vi "TSM DCPower Initialize Sessions.vi"(0 "TSM context":T2, 5 "Power Line Frequency":T1=60.0 caption="Power Line Frequency (60Hz)" items=["50 Hertz"=50.0, "60 Hertz"=60.0], 7 "Use Measure Multiple for Auto Measurement Mode? (T)":bool=TRUE) -> (15 "error out":errorcluster)   [LabVIEW 2020]
uses:
  <vilib>/NI_TestStand_SemiconductorModule/NI_TestStand_Semiconductor_Module.lvlibp/PinMap/General/SemiconductorModuleContext.ctl
  <instrlib>/niDCPower/nidcpower.llb/niDCPower Power Line Frequency.ctl
  <instrlib>/niDCPower/nidcpower.llb/niDCPower Sense.ctl
  SSC DCPower/Measure/SSC DCPower Debug Global.vi
  <vilib>/regexp/Match Regular Expression.xnode
  <vilib>/NI_TestStand_SemiconductorModule/NI_TestStand_Semiconductor_Module.lvlibp
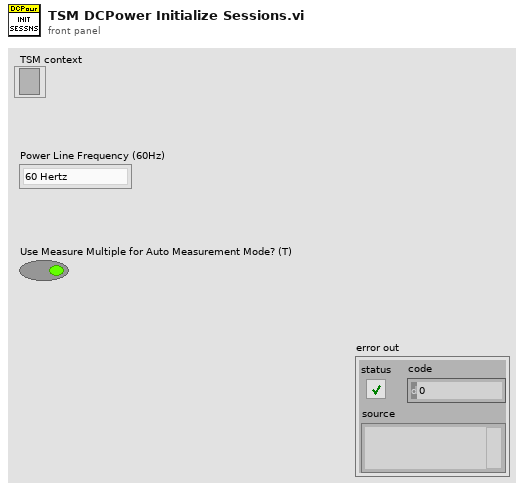
[diagram p1: front panel]
types:
  T1 = typedef "niDCPower Power Line Frequency.ctl" = dbl
  T2 = typedef "NI_TestStand_Semiconductor_Module.lvlibp/SemiconductorModuleContext.ctl" = refnum<k7>
  T3 = typedef "niDCPower Sense.ctl" = i32
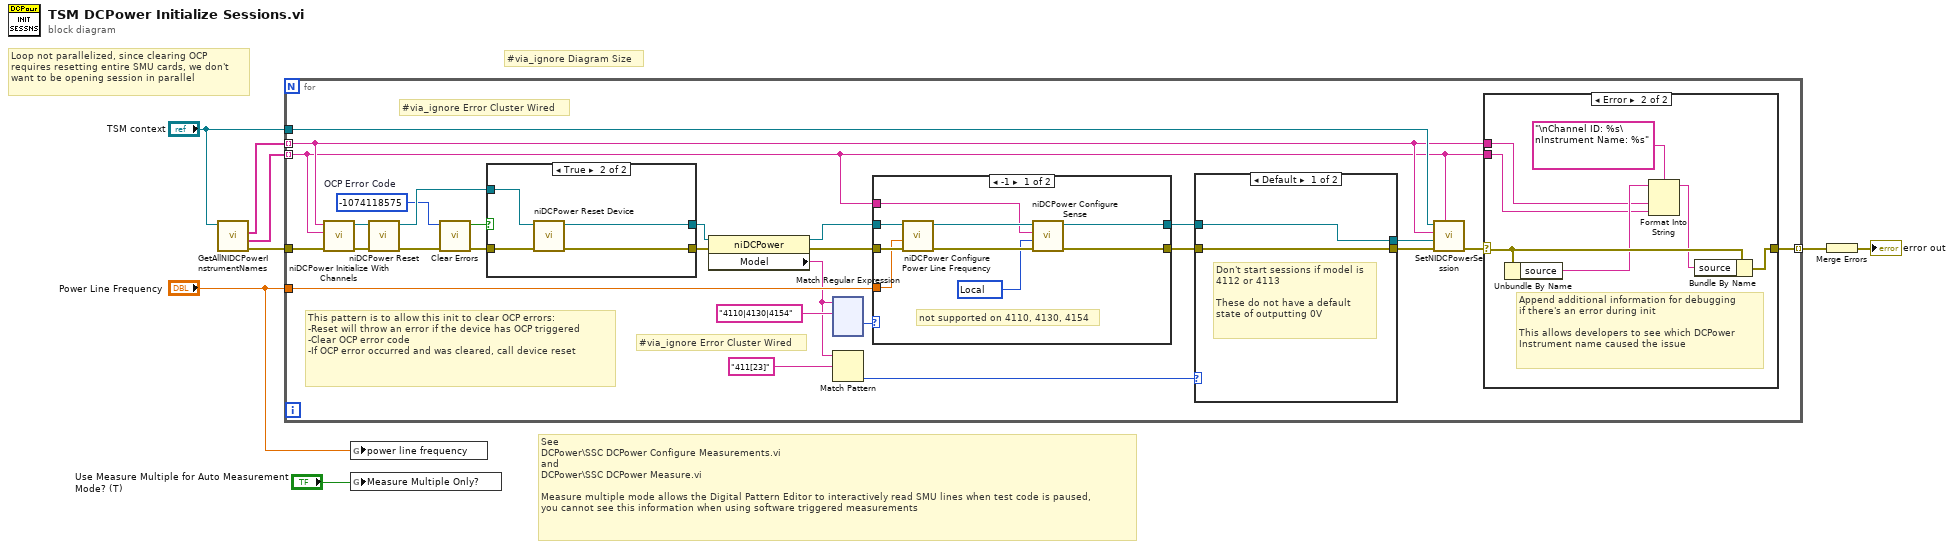
[diagram p0: block diagram]
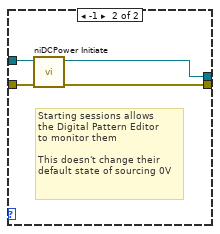
[diagram p5: hidden frame]
diagram:
  # "See \nDCPower\\SSC DCPower Configure Measurements.vi\nand\nDCPower\\SSC DCPower Measure.vi\n\nMeasure multiple mode allows the Digital Pattern Editor to interactively read SMU lines when test code is paused,\nyou cannot see this information when using software triggered measurements"
  # "#via_ignore Diagram Size"
  # "Loop not parallelized, since clearing OCP requires resetting entire SMU cards, we don't want to be opening session in parallel"
  n1 = call <vilib>:"GetAllNIDCPowerInstrumentNames.vi"("Semiconductor Module Context"="TSM context") -> ("error out"=w5:errorcluster, "Channel Ids"=w8:string[], "Instrument Names"=w4:string[])  [unwired: 7 in, 1 out]
  n2 = for {
    tunnel: w4 -> [w10] mode=indexing
    tunnel: w8 -> [w9] mode=indexing
    tunnel: "TSM context" -> [w35]
    tunnel: "Power Line Frequency" -> [w25]
    tunnel: w5 -> [w19]
    tunnel: [w11] -> w6 mode=indexing
    w14 = -1074118575  # OCP Error Code
    # "#via_ignore Error Cluster Wired"
    # "This pattern is to allow this init to clear OCP errors:\n-Reset will throw an error if the device has OCP triggered\n-Clear OCP error code\n-If OCP error occurred and was cleared, call device reset"
    # "#via_ignore Error Cluster Wired"
    n3 = call <instrlib>:"niDCPower Initialize With Channels.vi"("error in (no error)"=w19, "channels"=w9, "resource name"=w10) -> ("error out"=w31:errorcluster, "instrument handle out"=w17:refnum<k15>)  [unwired: 7 in]
    n4 = call <instrlib>:"niDCPower Reset.vi"("error in (no error)"=w31, "instrument handle"=w17) -> ("error out"=w18:errorcluster, "instrument handle out"=w16:refnum<k15>)  [unwired: 8 in]
    n5 = call <vilib>:"Clear Errors.vi"("error in (no error)"=w18, "specific error code to clear (0: all)"=w14) -> ("error out"=w15:errorcluster, "specific error cleared?"=w13:bool)  [unwired: 4 in]
    n6 = case shown="True" w13 {
      tunnel: [w44 w49] -> w21
      tunnel: w16 -> [w45 w46]
      tunnel: [w45 w48] -> w20
      tunnel: w15 -> [w44 w47]
      frame False {
      }
      frame True {
        n7 = call <instrlib>:"niDCPower Reset Device.vi"("error in (no error)"=w47, "instrument handle"=w46) -> ("error out"=w49:errorcluster, "instrument handle out"=w48:refnum<k15>)  [unwired: 8 in]
      }
    }
    n8 = property class="niDCPower"(reference=w20, error in=w21) -> (reference out=w27:refnum<k15>, error out=w30:errorcluster, "Model"=w22:string)
    n9 = xnode "Match Regular Expression"("input string"=w22, "regular expression"="4110|4130|4154") -> ("offset past match"=w23:i32)  [unwired: 4 in, 4 out]
    n10 = Match Pattern(string=w22, regular expression="411[23]") -> (offset past match=w29:i32)  [unwired: 1 in, 3 out]
    n11 = case shown="-1" w23 {
      tunnel: w30 -> [w172 w174]
      tunnel: [w168 w174] -> w28
      tunnel: w27 -> [w170 w173]
      tunnel: [w166 w173] -> w26
      tunnel: w25 -> [w169 _]
      tunnel: w9 -> [w165 _]
      frame -1 {
        w164 = T3 1008 items=["Local"=1008, "Remote"=1009] ("sense")
        # "not supported on 4110, 4130, 4154"
        n12 = call <instrlib>:"niDCPower Configure Power Line Frequency.vi"("error in (no error)"=w172, "power line frequency"=w169, "instrument handle"=w170) -> ("error out"=w171:errorcluster, "instrument handle out"=w167:refnum<k15>)  [unwired: 7 in]
        n13 = call <instrlib>:"niDCPower Configure Sense.vi"("error in (no error)"=w171, "sense"=w164, "channel name"=w165, "instrument handle"=w167) -> ("error out"=w168:errorcluster, "instrument handle out"=w166:refnum<k15>)  [unwired: 6 in]
      }
      frame Default {
      }
    }
    n14 = case shown="Default" w29 {
      tunnel: [w176 w180] -> w34
      tunnel: [w175 w179] -> w33
      tunnel: w28 -> [w175 w178]
      tunnel: w26 -> [w176 w177]
      frame Default {
        # "Don't start sessions if model is\n4112 or 4113\n\nThese do not have a default\nstate of outputting 0V"
      }
      frame -1 {
        # "Starting sessions allows\nthe Digital Pattern Editor\nto monitor them\n\nThis doesn't change their\ndefault state of sourcing 0V"
        n15 = call <instrlib>:"niDCPower Initiate.vi"("error in (no error)"=w178, "instrument handle"=w177) -> ("error out"=w179:errorcluster, "instrument handle out"=w180:refnum<k15>)  [unwired: 8 in]
      }
    }
    n16 = call <vilib>:"SetNIDCPowerSession.vi"("Channel Id"=w9, "error in (no error)"=w33, "Instrument Session"=w34, "Instrument Name"=w10, "Semiconductor Module Context"=w35) -> ("error out"=w12:errorcluster)  [unwired: 5 in, 1 out]
    n17 = case shown="Error" w12 {
      selector: w12 -> [w36 w43]
      tunnel: [w36 w42] -> w11
      tunnel: w10 -> [_ w38]
      tunnel: w9 -> [_ w37]
      frame No Error {
      }
      frame Error {
        # "Append additional information for debugging\nif there's an error during init\n\nThis allows developers to see which DCPower\nInstrument name caused the issue"
        n18 = Unbundle By Name(w43) -> ("source"=w41:string)
        n19 = Format Into String(format string="\nChannel ID: %s\nInstrument Name: %s", initial string=w41, w38, w37) -> (resulting string=w40:string)  [unwired: 1 in, 1 out]
        n20 = Bundle By Name(cluster=w43, "source"=w40) -> (w42:errorcluster)
      }
    }
  }
  n21 = global write "SSC DCPower Debug Global.vi" "power line frequency"("Power Line Frequency") -> ()
  n22 = global write "SSC DCPower Debug Global.vi" "Measure Multiple Only?"("Use Measure Multiple for Auto Measurement Mode? (T)") -> ()
  n23 = Merge Errors(w6) -> (→"error out":errorcluster)
